vi "scan keypad.vi"(8 "error in (no error)":errorcluster, 11 "keypad ref":T1={"column drivers"={"myRIO Reference"={"myRIO Model"=enum."Unknown", "myRIO Hardware Reference"={"Generic FPGA Reference"=refnum, "Allow multiple opens"=FALSE}}, "DIO Channels List"=[]}, "row drivers"={"myRIO Reference"={"myRIO Model"=enum."Unknown", "myRIO Hardware Reference"={"Generic FPGA Reference"=refnum, "Allow multiple opens"=FALSE}}, "DIO Channels List"=[]}, "pull downs"=FALSE, "timeout [ms]"=4294967295}) -> (0 "error out":errorcluster, 2 "keypad code":i32, 3 "keypad ref out":T1={"column drivers"={"myRIO Reference"={"myRIO Model"=enum."Unknown", "myRIO Hardware Reference"={"Generic FPGA Reference"=refnum, "Allow multiple opens"=FALSE}}, "DIO Channels List"=[]}, "row drivers"={"myRIO Reference"={"myRIO Model"=enum."Unknown", "myRIO Hardware Reference"={"Generic FPGA Reference"=refnum, "Allow multiple opens"=FALSE}}, "DIO Channels List"=[]}, "pull downs"=FALSE, "timeout [ms]"=4294967295})   [LabVIEW 2013]
uses:
  keypad references.ctl
  <vilib>/myRIO/Instrument Drivers/Onboard IO/DIO/typedefs/DIO Reference.ctl
  <vilib>/myRIO/Common/Instrument Driver Framework/Utilities/typedefs/myRIO Generic Hardware Reference.ctl
  <vilib>/myRIO/Common/Instrument Driver Framework/Utilities/typedefs/Hardware Version Enum.ctl
  <vilib>/myRIO/Common/Instrument Driver Framework/Utilities/typedefs/myRIO v1.0 Reference.ctl
  <vilib>/myRIO/Common/Instrument Driver Framework/Utilities/typedefs/Generic FPGA Reference.ctl
  <vilib>/myRIO/Common/Instrument Driver Framework/myRIO v1.0/DIO/typedefs/DIO Channels List.ctl
  <vilib>/myRIO/Common/Instrument Driver Framework/myRIO v1.0/DIO/typedefs/DIO Channels Enum.ctl
  <vilib>/Utility/error.llb/Error Cluster From Error Code.vi
  <vilib>/myRIO/Common/Instrument Driver Framework/myRIO v1.0/DIO/vis/myRIO v1.0 Read DIO.vi
  <vilib>/myRIO/Common/Instrument Driver Framework/myRIO v1.0/DIO/vis/myRIO v1.0 Write DIO.vi
  <vilib>/myRIO/Instrument Drivers/Onboard IO/DIO/DIO.lvlib
panel:
  # "Scan keypad"
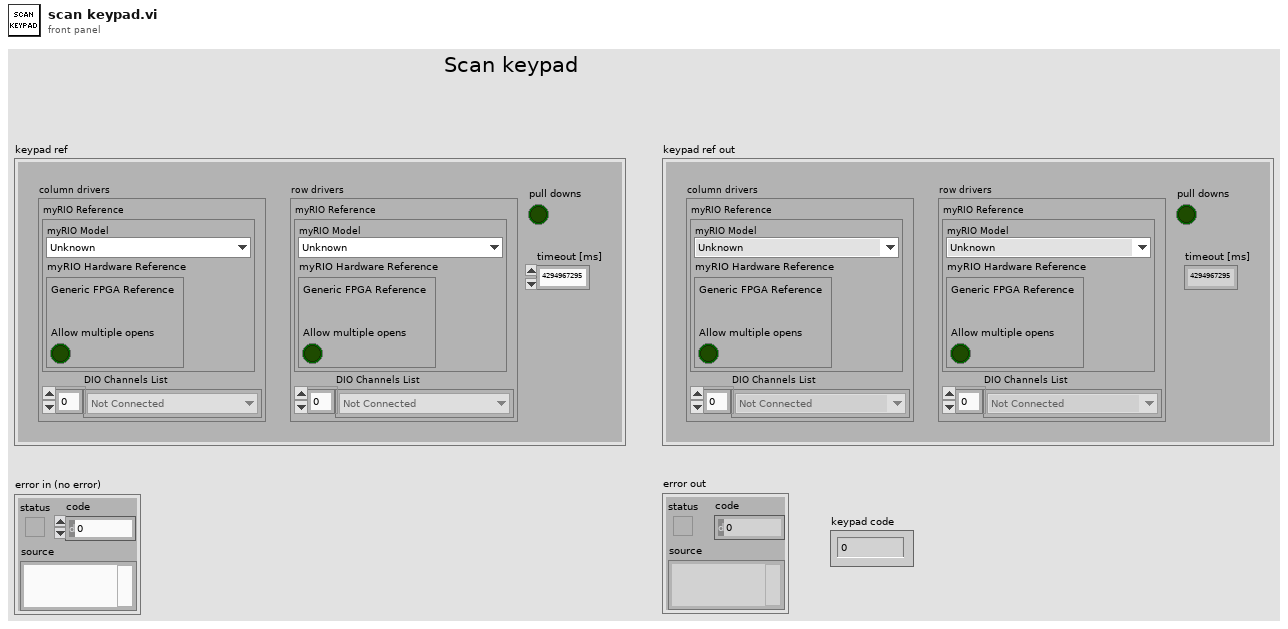
[diagram p1: front panel]
types:
  T1 = typedef "keypad references.ctl" = cluster{"column drivers":T2, "row drivers":T2, "pull downs":bool, "timeout [ms]":u32}
  T2 = typedef "DIO.lvlib/DIO Reference.ctl" = cluster{"myRIO Reference":T3, "DIO Channels List":T7}
  T3 = typedef "myRIO Generic Hardware Reference.ctl" = cluster{"myRIO Model":T4, "myRIO Hardware Reference":T5}
  T4 = typedef "Hardware Version Enum.ctl" = enum16{"Unknown", "myRIO-1900", "myRIO-1950"}
  T5 = typedef "myRIO v1.0 Reference.ctl" = cluster{"Generic FPGA Reference":T6, "Allow multiple opens":bool}
  T6 = typedef "Generic FPGA Reference.ctl" = refnum<k20>
  T7 = typedef "DIO Channels List.ctl" = T8[]
  T8 = typedef "DIO Channels Enum.ctl" = enum16{"Not Connected", "C/DIO0", "C/DIO1", "C/DIO2", "C/DIO3", "C/DIO4", "C/DIO5", "C/DIO6", "C/DIO7", "A/DIO0", "A/DIO1", "A/DIO2", "A/DIO3", "A/DIO4", "A/DIO5", "A/DIO6", "A/DIO7", "A/DIO8", "A/DIO9", "A/DIO10", "A/DIO11", "A/DIO12", "A/DIO13", "A/DIO14", "A/DIO15", "B/DIO0", "B/DIO1", "B/DIO2", "B/DIO3", "B/DIO4", "B/DIO5", "B/DIO6", "B/DIO7", "B/DIO8", "B/DIO9", "B/DIO10", "B/DIO11", "B/DIO12", "B/DIO13", "B/DIO14", "B/DIO15", "LED0", "LED1", "LED2", "LED3", "Button0"}
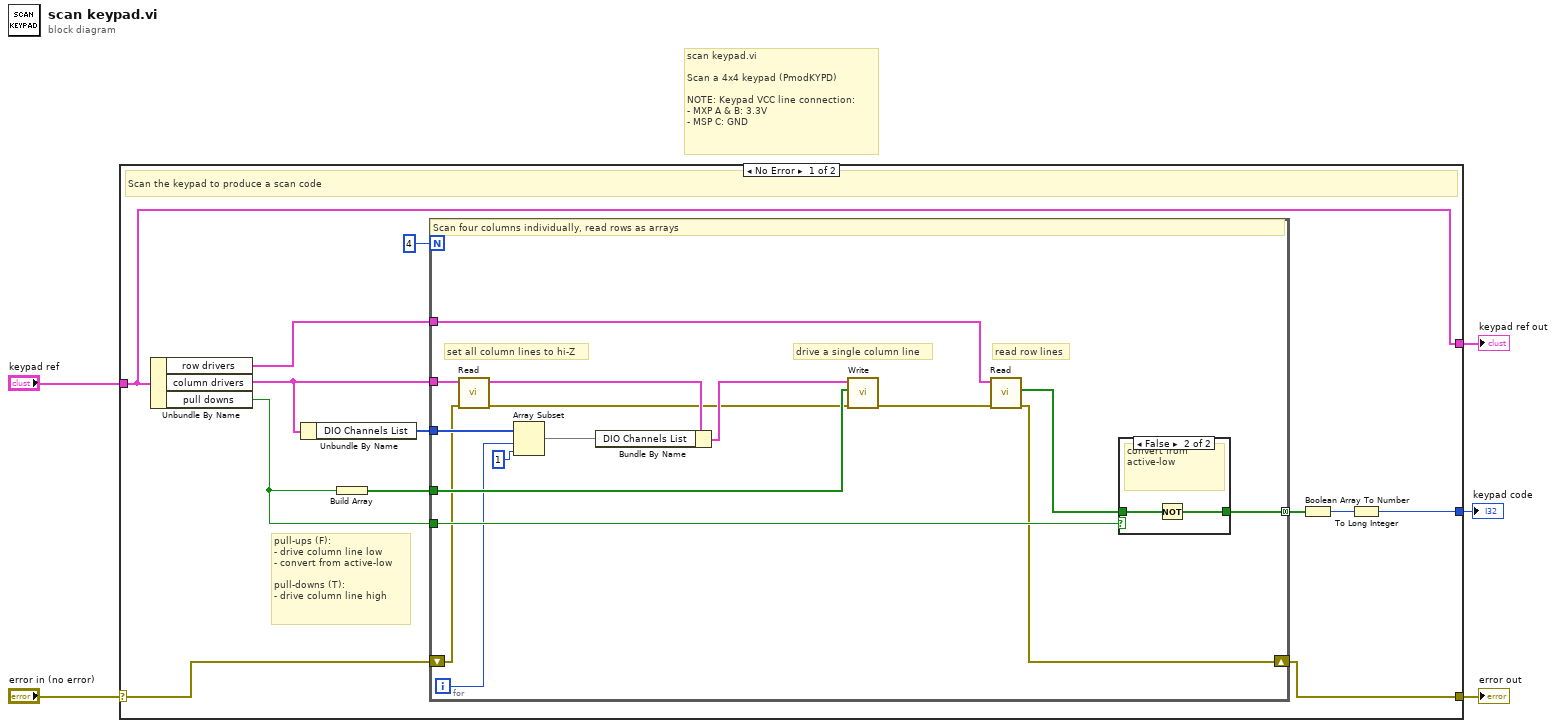
[diagram p0: block diagram]
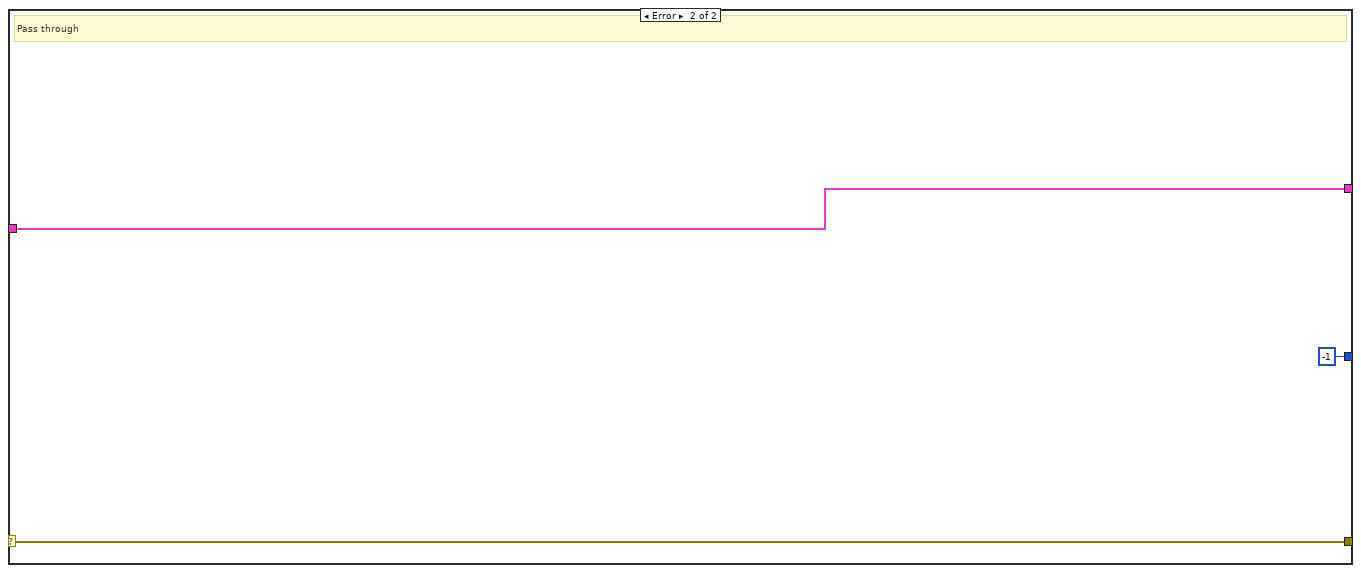
[diagram p3: hidden frame]
diagram:
  # "scan keypad.vi\n\nScan a 4x4 keypad (PmodKYPD)\n\nNOTE: Keypad VCC line connection:\n- MXP A & B: 3.3V\n- MSP C: GND"
  n1 = case shown="No Error" "error in (no error)" {
    selector: "error in (no error)" -> [w12 w39]
    tunnel: [w17 w39] -> w4
    tunnel: [w13 -1] -> w1
    tunnel: [w6 w37] -> w2
    tunnel: "keypad ref" -> [w6 w37]
    frame No Error {
      # "pull-ups (F):\n- drive column line low\n- convert from active-low\n\npull-downs (T):\n- drive column line high"
      # "Scan the keypad to produce a scan code"
      n2 = Unbundle By Name(w6) -> ("row drivers"=w7:T2, "column drivers"=w9:T2, "pull downs"=w10:bool)
      n3 = Unbundle By Name(w9) -> ("DIO Channels List"=w8:T7)
      n4 = Build Array "Build Array"(w10) -> (w11:bool[])
      n5 = for {
        N: 4 -> [_]
        shift-right: [w18] -> w17
        shift-left: w12 -> [w22]
        tunnel: [w33] -> w15 mode=concatenating
        tunnel: w11 -> [w32]
        tunnel: w10 -> [w30]
        tunnel: w9 -> [w29]
        tunnel: w8 -> [w28]
        tunnel: w7 -> [w19]
        i -> [w27]
        # "set all column lines to hi-Z"
        # "read row lines"
        # "drive a single column line"
        # "Scan four columns individually, read rows as arrays"
        n6 = call <vilib>:"Read.vi"("error in (no error)"=w22, "DIO Ref In"=w29) -> ("error out"=w21:errorcluster, "DIO Ref Out"=w26:T2)  [unwired: 7 in, 1 out]
        n7 = Array Subset "Array Subset"(array=w28, index=w27, length=1) -> (w24:T7)
        n8 = Bundle By Name(cluster=w26, "DIO Channels List"=w24) -> (w23:T2)
        n9 = call <vilib>:"Write.vi"("error in (no error)"=w21, "Values"=w32, "DIO Ref In"=w23) -> ("error out"=w20:errorcluster)  [unwired: 6 in, 1 out]
        n10 = call <vilib>:"Read.vi"("error in (no error)"=w20, "DIO Ref In"=w19) -> ("error out"=w18:errorcluster, "Values"=w31:bool[])  [unwired: 7 in, 1 out]
        n11 = case shown="False" w30 {
          tunnel: [w34 w36] -> w33
          tunnel: w31 -> [w34 w35]
          frame True {
            # "already active-high"
          }
          frame False {
            # "convert from active-low"
            n12 = Not(x=w35) -> (.not. x?=w36:bool[])
          }
        }
      }
      n13 = Boolean Array To Number(Boolean array=w15) -> (number=w14:u32)
      n14 = To Long Integer(number=w14) -> (32bit integer=w13:i32)
    }
    frame Error {
      # "Pass through"
    }
  }
  "error out" <- w4
  "keypad ref out" <- w2
  "keypad code" <- w1
